vi "get&set FileFormat.vi"(6 "Get/Set? (Set)":bool=TRUE, 8 "error in (no error)":errorcluster, 10 "FileFormat":i32(ring)=1448157312 items=["Raw"=1448157312, "Gzip"=1448157313, "Tiff"=1448157314, "Jpeg"=1448157315, "Bmp"=1448157316, "Bir"=1448157317, "Toshiba"=1448157318, "Shimadzu"=1448157319, "Pnm"=1448157320, "Jpeg2"=1448157321, "Yxlon"=1448157322, "Hdf"=1448157323, "Dicom"=1448157324, "Imtec"=1448157325, "Aracor"=1448157326, "Fhg"=1448157327], 11 "VGS_VolumeDescriptor+File in":refnum<class "VGS_VolumeDescriptor+File.lvclass">) -> (0 "error out":errorcluster, 2 "FileFormat":i32(ring)=1448157312 items=["Raw"=1448157312, "Gzip"=1448157313, "Tiff"=1448157314, "Jpeg"=1448157315, "Bmp"=1448157316, "Bir"=1448157317, "Toshiba"=1448157318, "Shimadzu"=1448157319, "Pnm"=1448157320, "Jpeg2"=1448157321, "Yxlon"=1448157322, "Hdf"=1448157323, "Dicom"=1448157324, "Imtec"=1448157325, "Aracor"=1448157326, "Fhg"=1448157327], 3 "VGS_VolumeDescriptor+File out":refnum<class "VGS_VolumeDescriptor+File.lvclass">)   [LabVIEW 2022 SP3, in "LV_VGS.lvlib" / "VGS_VolumeDescriptor+File.lvclass"]
doc: "<B>Defines physical position of a single slice file. </B>\n\nDefines the relative physical position of a single slice file. Use this function if the file represents a single xy-slice (z-size is 1).\n\nThis function is equivalent to calling setPositionList() with a list of size 1. See setPositionList() for details. \n\n<B>bool VGS::Project::Interop::VolumeDescriptor::File::setPositionList ( List< float >^ positionList ) </B>\n\nDefines physical positions of the file's slices. \n\nDefines the relative physical position of all the slices represented by this file. Use this function to define non-equidistant slices: normally, the slice distance is determined globally by the z-component of VolumeDescriptor.Resolution, i.e. all given xy-slices are the same distance apart. If your scanned data has varying slice distances, however, you can define a kind of physical position (in mm) for each slice. These distances will then be used instead of the z-resolution value, which will be ignored.\n\n You cannot \"mix\" specifications: if you specify a position list, you must do it for all files in the VolumeDescriptor, and each file must specify as many positions as its z-size indicates! \n Optional definition. The default value is an empty list."
uses:
  VGS_VolumeDescriptor+File.lvclass
  VGS_VolumeDescriptor+File.lvclass/VGS_VolumeDescriptor+File.ctl
  C:/Users/Andrey/Desktop/hajo/LV_VGS/vgs_project.dll
  vgs_project.dll
panel:
  # "-Set\n-Get"
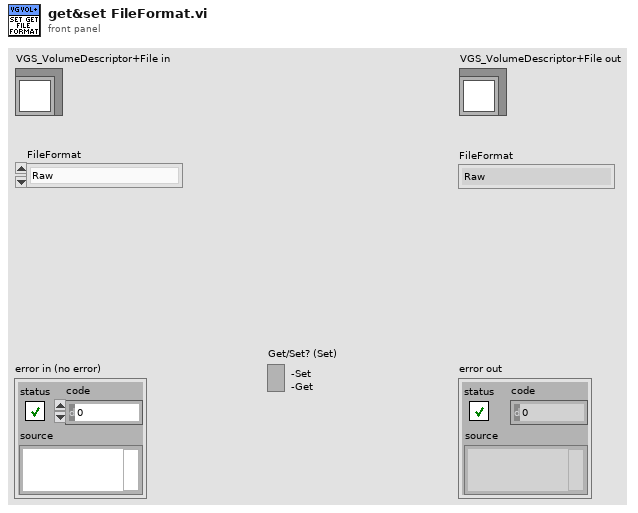
[diagram p1: front panel]
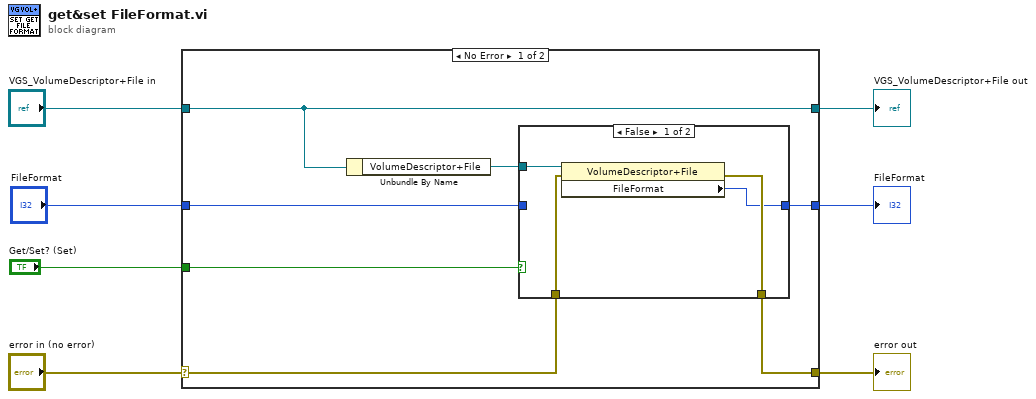
[diagram p0: block diagram]
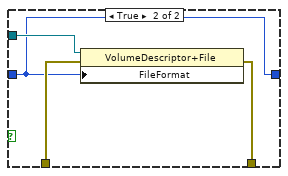
[diagram p2: hidden frame]
diagram:
  n1 = case shown="No Error" "error in (no error)" {
    selector: "error in (no error)" -> [w12 w25]
    tunnel: [w11 w25] -> w6
    tunnel: [w14 w24] -> w4
    tunnel: "VGS_VolumeDescriptor+File in" -> [w14 w24]
    tunnel: "Get/Set? (Set)" -> [w10 _]
    tunnel: "FileFormat" -> [w9 w23]
    tunnel: [w8 w23] -> w1
    frame No Error {
      n2 = Unbundle By Name(w14) -> ("VolumeDescriptor+File"=w13:refnum<k24>)
      n3 = case shown="False" w10 {
        tunnel: w13 -> [w18 w20]
        tunnel: w12 -> [w17 w22]
        tunnel: [w16 w21] -> w11
        tunnel: w9 -> [_ w19]
        tunnel: [w15 w19] -> w8
        frame False {
          n4 = property class="VolumeDescriptor+File"(reference=w18, error in=w17) -> (error out=w16:errorcluster, "FileFormat"=w15:i32)  [unwired: 1 out]
        }
        frame True {
          n5 = property class="VolumeDescriptor+File"(reference=w20, error in=w22, "FileFormat"=w19) -> (error out=w21:errorcluster)  [unwired: 1 out]
        }
      }
    }
    frame Error {
    }
  }
  "error out" <- w6
  "VGS_VolumeDescriptor+File out" <- w4
  "FileFormat" <- w1
